vi "Setup Reply Queue.vi"(8 "error in (no error)":errorcluster) -> (0 "error out":errorcluster, 3 "Queue out":refnum<queue>)   [LabVIEW 2015, in "Command Handler.lvlib" / "Command Handler.lvclass"]
uses:
  Command Handler.lvclass
  Type Defs/Command Handler Data.ctl
  Type Defs/Event Cluster.ctl
  Command Parent/Command.lvclass
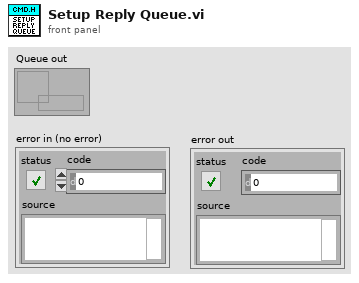
[diagram p1: front panel]
types:
  T1 = typedef "Command Handler.lvlib/Command Handler.lvclass/Event Cluster.ctl" = cluster{"Error Event":refnum<user-event>, "Command Done Event":refnum<user-event>, "Stopping Event":refnum<user-event>, "Data Update Event":refnum<user-event>}
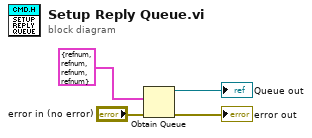
[diagram p0: block diagram]
diagram:
  n1 = Obtain Queue(element data type=T1 {"Error Event"=refnum, "Command Done Event"=refnum, "Stopping Event"=refnum, "Data Update Event"=refnum} ("Actor Events"), error in (no error)="error in (no error)") -> (queue out=→"Queue out":refnum<queue>, error out=→"error out":errorcluster)  [unwired: 3 in, 1 out]
